vi "Send Command.vi"() -> ()   [LabVIEW 2009]
panel:
  in  "write buffer":string
  in  "error in (no error)":errorcluster
  out "error out":errorcluster
  out "VISA resource name out":refnum<visa-resource-name>
  in  "VISA resource name":refnum<visa-resource-name>
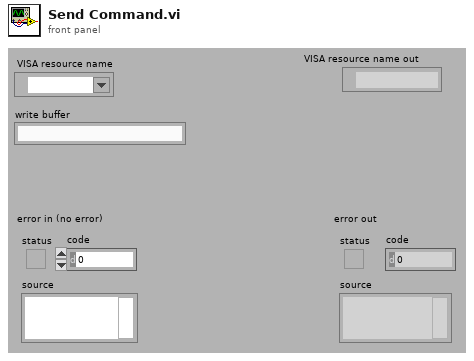
[diagram p1: front panel]
types:
  T1 = typedef "Semaphore RefNum" = refnum<k1>
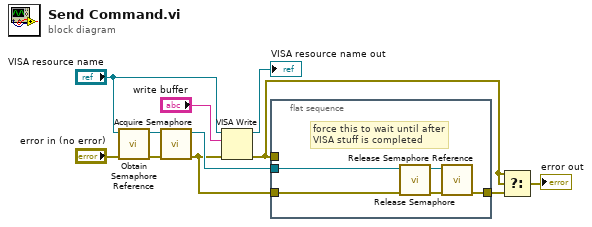
[diagram p0: block diagram]
diagram:
  n1 = call <vilib>:"Obtain Semaphore Reference.vi"("error in (no error)"="error in (no error)", "name (unnamed)"="VISA resource name") -> ("error out"=w9:errorcluster, "semaphore"=w10:T1)  [unwired: 1 in, 3 out]
  n2 = call <vilib>:"Acquire Semaphore.vi"("error in (no error)"=w9, "semaphore"=w10) -> ("error out"=w5:errorcluster, "semaphore out"=w7:T1)  [unwired: 1 in, 3 out]
  n3 = VISA Write(VISA resource name="VISA resource name", write buffer="write buffer", error in (no error)=w5) -> (VISA resource name out=→"VISA resource name out":refnum<visa-resource-name>, error out=w1:errorcluster)  [unwired: 1 out]
  n4 = flat-sequence {
    tunnel: w7 -> [w16]
    tunnel: [w13] -> w4
    tunnel: w1 -> [_]
    tunnel: w5 -> [w12]
    frame #0 {
      # "force this to wait until after \nVISA stuff is completed"
      n5 = call <vilib>:"Release Semaphore.vi"("error in (no error)"=w12, "semaphore"=w16) -> ("error out"=w14:errorcluster, "semaphore out"=w15:T1)  [unwired: 4 out]
      n6 = call <vilib>:"Release Semaphore Reference.vi"("error in (no error)"=w14, "semaphore"=w15) -> ("error out"=w13:errorcluster)  [unwired: 9 out]
    }
  }
  n7 = Select(t=w1, s=w1, f=w4) -> (s? t:f=→"error out":errorcluster)
